vi "DN4_UpDownCounter_GetValue.vi"(3 "reset updown count?":bool, 4 "error in (no error)":errorcluster, 5 "Task ID":u32) -> (0 "updown count":i32, 1 "error out":errorcluster, 2 "Task ID out":u32)   [LabVIEW 2009]
uses:
  Windows/System32/AdvLvDaq.dll
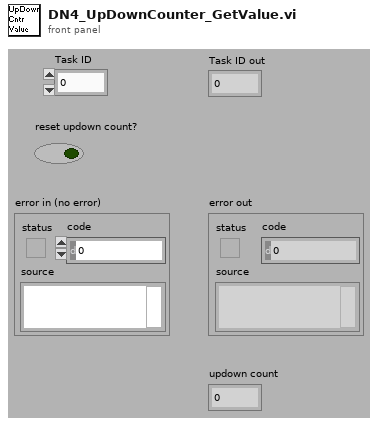
[diagram p1: front panel]
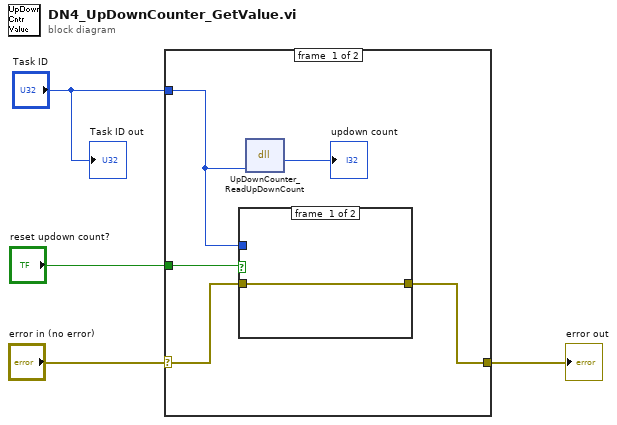
[diagram p0: block diagram]
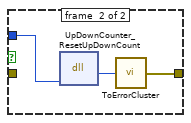
[diagram p2: hidden frame]
diagram:
  n1 = case shown="No Error" "error in (no error)" {
    selector: "error in (no error)" -> [w5 w14]
    tunnel: [w6 w14] -> w3
    tunnel: "Task ID" -> [w7 _]
    tunnel: "reset updown count?" -> [w8 _]
    frame #0 {
      n2 = case shown="True" w8 {
        tunnel: w7 -> [_ w13]
        tunnel: [w10 w11] -> w6
        tunnel: w5 -> [w10 _]
        frame #0 {
        }
        frame #1 {
          n3 = dll-call lib="C:/Windows/System32/AdvLvDaq.dll" fn="UpDownCounter_ResetUpDownCount"("taskID"=w13) -> ("error code"=w12:i32)  [unwired: 4 in, 2 out]
          n4 = call <userlib>:"ToErrorCluster.vi"("error code"=w12) -> ("error out"=w11:errorcluster)
        }
      }
      n5 = dll-call lib="C:/Windows/System32/AdvLvDaq.dll" fn="UpDownCounter_ReadUpDownCount"("taskID"=w7) -> ("updownCount"=→"updown count":i32)  [unwired: 4 in, 2 out]
    }
    frame #1 {
    }
  }
  "error out" <- w3
  "Task ID out" <- "Task ID"
